vi "CommandWriteandReturn.vi"(8 "error in (no error)":errorcluster, 10 "Write Buffer":string, 11 "VISA resource name":refnum<visa-resource-name>="LitePoint_IQxstream") -> (0 "error out":errorcluster, 1 "array":dbl[](array[numeric]) format="%.2g", 2 "read buffer":string, 3 "VISA resource name out":refnum<visa-resource-name>)   [LabVIEW 2020, in "LitePoints.lvlib"]
uses:
  LitePoints.lvlib
panel:
  out "return count":u32
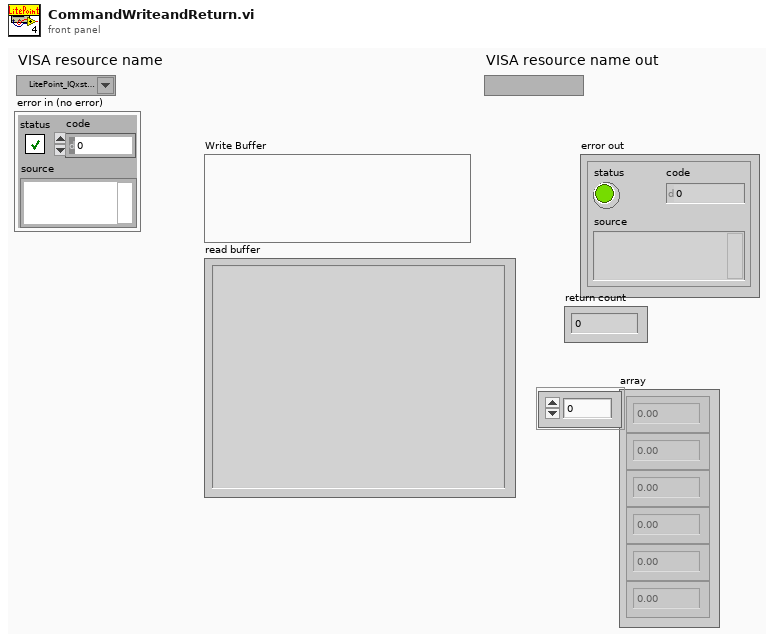
[diagram p1: front panel]
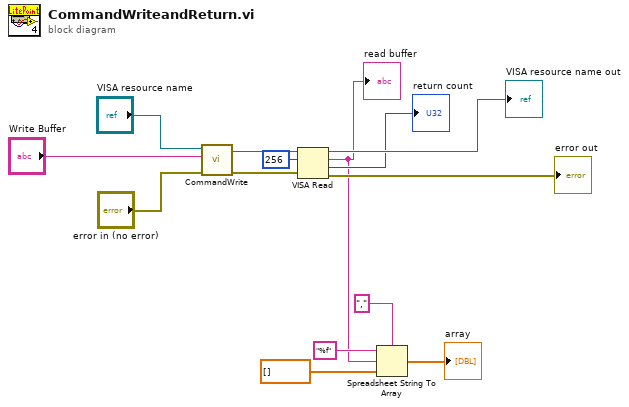
[diagram p0: block diagram]
diagram:
  n1 = call "CommandWrite.vi"("error in (no error)"="error in (no error)", "Write Buffer"="Write Buffer", "VISA resource name"="VISA resource name") -> ("error out"=w11:errorcluster, "VISA resource name out"=w12:refnum<visa-resource-name>)  [unwired: 7 in]
  n2 = VISA Read(VISA resource name=w12, byte count=u32 256, error in (no error)=w11) -> (VISA resource name out=→"VISA resource name out":refnum<visa-resource-name>, read buffer=w1:string, return count=→"return count":u32, error out=→"error out":errorcluster)
  "read buffer" <- w1
  n3 = Spreadsheet String To Array(delimiter (Tab)="," ("spreadsheet string"), format string="%f", spreadsheet string=w1, array type (2D Dbl)=dbl[] []) -> (array=→"array":dbl[])
